vi "AOC.vi"(1 "radius":dbl) -> (0 "output":dbl)   [LabVIEW 2017]
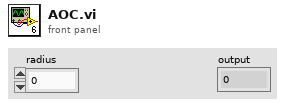
[diagram p1: front panel]
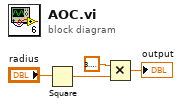
[diagram p0: block diagram]
diagram:
  n1 = Square(x="radius") -> (x^2=w3:dbl)
  n2 = Multiply(x=3.141592653589793, y=w3) -> (x*y=→"output":dbl)
